vi "xy to direction.vi"(0 "Angle in":T1 items=["0", "45", "90", "135", "180", "225", "270", "315", "360"], 1 "stop":bool, 3 "Next X":i16, 4 "Next Y":i16, 5 "Start X":i16, 6 "Start Y":i16) -> (2 "Angle out":T1 items=["0", "45", "90", "135", "180", "225", "270", "315", "360"])   [LabVIEW 2014]
uses:
  Controls/Direction enum.ctl
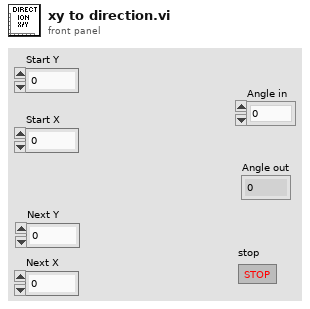
[diagram p1: front panel]
types:
  T1 = typedef "Direction enum.ctl" = u16
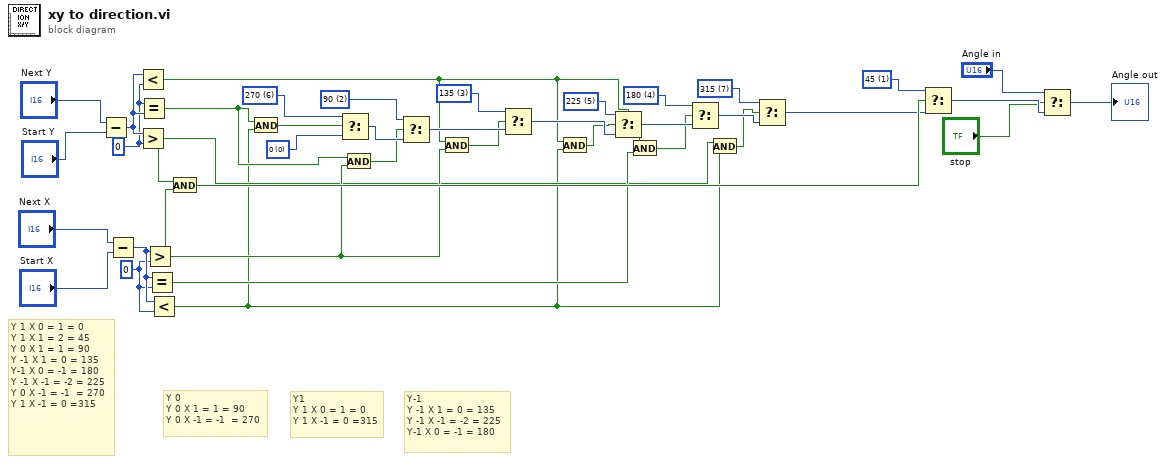
[diagram p0: block diagram]
diagram:
  w10 = T1 7 items=["0", "45", "90", "135", "180", "225", "270", "315", "360"] ("Ring")
  w15 = T1 4 items=["0", "45", "90", "135", "180", "225", "270", "315", "360"] ("Ring")
  w17 = T1 5 items=["0", "45", "90", "135", "180", "225", "270", "315", "360"] ("Ring")
  w20 = T1 3 items=["0", "45", "90", "135", "180", "225", "270", "315", "360"] ("Ring")
  w27 = T1 2 items=["0", "45", "90", "135", "180", "225", "270", "315", "360"] ("Ring")
  w29 = T1 6 items=["0", "45", "90", "135", "180", "225", "270", "315", "360"] ("Ring")
  w30 = T1 0 items=["0", "45", "90", "135", "180", "225", "270", "315", "360"] ("Ring")
  w35 = T1 1 items=["0", "45", "90", "135", "180", "225", "270", "315", "360"] ("Ring")
  w33 = i16 0 ("y")
  w31 = i16 0 ("y")
  # "Y-1\nY -1 X 1 = 0 = 135\nY -1 X -1 = -2 = 225\nY-1 X 0 = -1 = 180"
  # "Y1\nY 1 X 0 = 1 = 0\nY 1 X -1 = 0 =315"
  # "Y 0\nY 0 X 1 = 1 = 90\nY 0 X -1 = -1  = 270"
  # "Y 1 X 0 = 1 = 0\nY 1 X 1 = 2 = 45\nY 0 X 1 = 1 = 90\nY -1 X 1 = 0 = 135\nY-1 X 0 = -1 = 180\nY -1 X -1 = -2 = 225\nY 0 X -1 = -1  = 270\nY 1 X -1 = 0 =315"
  n1 = Subtract(x="Next Y", y="Start Y") -> (x-y=w32:i16)
  n2 = Subtract(x="Next X", y="Start X") -> (x-y=w34:i16)
  n3 = Less?(x=w32, y=w31) -> (x < y?=w12:bool)
  n4 = Greater?(x=w32, y=w31) -> (0:w9:bool)
  n5 = Equal?(x=w31, y=w32) -> (x = y?=w25:bool)
  n6 = Greater?(x=w34, y=w33) -> (0:w22:bool)
  n7 = Equal?(x=w34, y=w33) -> (x = y?=w13:bool)
  n8 = Less?(x=w34, y=w33) -> (x < y?=w8:bool)
  n9 = And(x=w9, y=w22) -> (x .and. y?=w36:bool)
  n10 = And(x=w25, y=w8) -> (x .and. y?=w26:bool)
  n11 = Select(t=w29, s=w26, f=w30) -> (s? t:f=w28:T1)
  n12 = And(x=w25, y=w22) -> (x .and. y?=w24:bool)
  n13 = Select(t=w27, s=w24, f=w28) -> (s? t:f=w23:T1)
  n14 = And(x=w12, y=w22) -> (x .and. y?=w21:bool)
  n15 = Select(t=w20, s=w21, f=w23) -> (s? t:f=w19:T1)
  n16 = And(x=w12, y=w8) -> (x .and. y?=w18:bool)
  n17 = Select(t=w17, s=w18, f=w19) -> (s? t:f=w16:T1)
  n18 = And(x=w12, y=w13) -> (x .and. y?=w14:bool)
  n19 = Select(t=w15, s=w14, f=w16) -> (s? t:f=w11:T1)
  n20 = And(x=w9, y=w8) -> (x .and. y?=w7:bool)
  n21 = Select(t=w10, s=w7, f=w11) -> (s? t:f=w6:T1)
  n22 = Select(t=w35, s=w36, f=w6) -> (s? t:f=w3:T1)
  n23 = Select(t="Angle in", s="stop", f=w3) -> (s? t:f=→"Angle out":T1)
